vi "Toggle Lift Piston.vi"   [LabVIEW 2019]
uses:
  <vilib>/Rock Robotics/WPI/Solenoid/WPI_SolenoidValue.ctl
  <vilib>/Rock Robotics/WPI/Solenoid/Deprecated/WPI_SolenoidGetBool.vi
  <vilib>/Rock Robotics/WPI/Solenoid/WPI_SolenoidSetEnum.vi
types:
  T1 = typedef "WPI_SolenoidValue.ctl" = enum16{"Off", "On", "Forward", "Reverse"}
  T2 = typedef "WPI_SolenoidDevRef.ctl" = cluster{"DevStatus":errorcluster, "Pneumatics Control Module":u8, "Forward Solenoid Channel":T3, "Reverse Solenoid Channel":T3}
  T3 = typedef "WPI_SolenoidChannel.ctl" = enum8{"Solenoid 0", "Solenoid 1", "Solenoid 2", "Solenoid 3", "Solenoid 4", "Solenoid 5", "Solenoid 6", "Solenoid 7", "Invalid"}
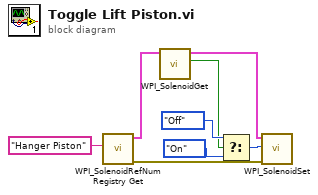
[diagram p0: block diagram]
diagram:
  n1 = call <vilib>:"WPI_SolenoidRefNum Registry Get.vi"("refnum name"="Hanger Piston") -> ("error out"=w7:errorcluster, "SolenoidDevRef"=w2:T2)  [unwired: 9 in]
  n2 = call-poly <vilib>:"WPI_SolenoidGet.vi"("SolenoidDevRef"=w2) -> ("Value"=w3:bool, "SolenoidDevRef"=w1:T2)  [unwired: 8 in, 1 out]
  n3 = Select(t=WPI_SolenoidValue."Off" ("Value"), s=w3, f=WPI_SolenoidValue."On" ("Value")) -> (s? t:f=w4:T1)
  n4 = call-poly <vilib>:"WPI_SolenoidSet.vi"("error in (no error)"=w7, "Value"=w4, "SolenoidDevRef"=w1) -> ()  [unwired: 7 in, 2 out]
